vi "Induction Range Bit Pack Parse.vi"(10 "Raw Data":string, 11 "Boolean array":bool[](array[boolean])) -> (3 "String":string)   [LabVIEW 2016]
uses:
  <vilib>/Utility/error.llb/whitespace.ctl
panel:
  out "Error Out":errorcluster
  in  "Error In":errorcluster
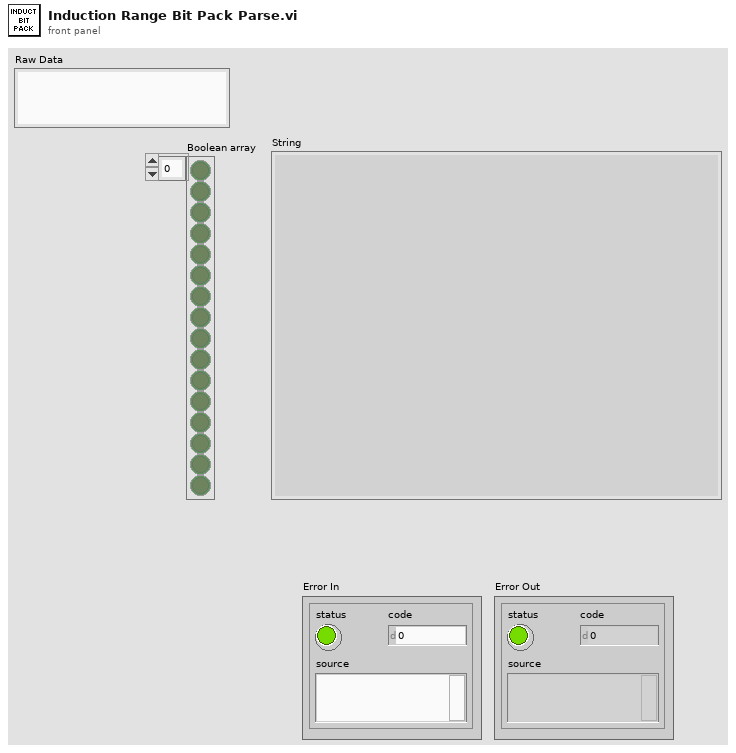
[diagram p1: front panel]
types:
  T1 = typedef "whitespace.ctl" = u16
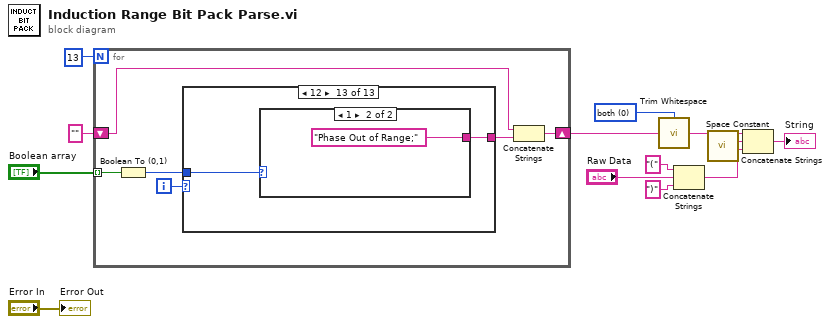
[diagram p0: block diagram]
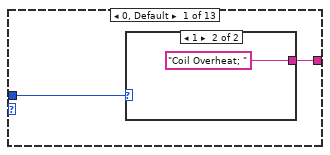
[diagram p2: hidden frame]
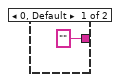
[diagram p3: hidden frame]
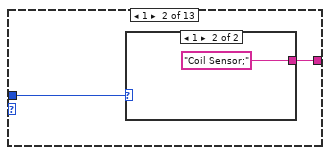
[diagram p4: hidden frame]
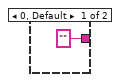
[diagram p5: hidden frame]
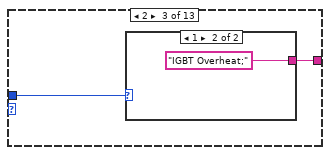
[diagram p6: hidden frame]
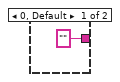
[diagram p7: hidden frame]
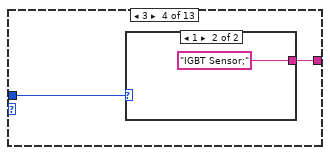
[diagram p8: hidden frame]
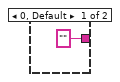
[diagram p9: hidden frame]
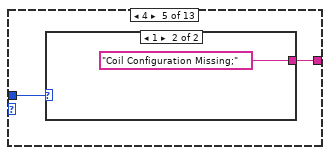
[diagram p10: hidden frame]
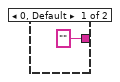
[diagram p11: hidden frame]
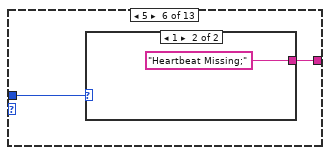
[diagram p12: hidden frame]
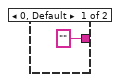
[diagram p13: hidden frame]
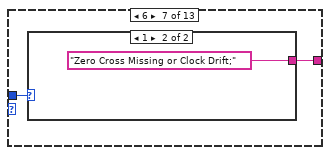
[diagram p14: hidden frame]
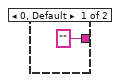
[diagram p15: hidden frame]
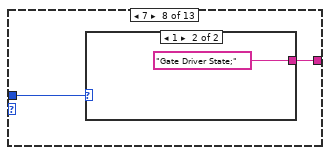
[diagram p16: hidden frame]
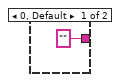
[diagram p17: hidden frame]
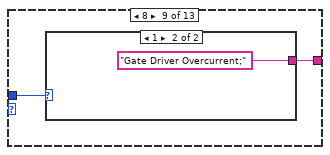
[diagram p18: hidden frame]
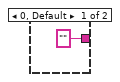
[diagram p19: hidden frame]
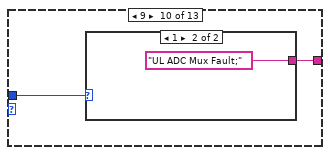
[diagram p20: hidden frame]
diagram:
  w8 = T1 0 items=["both", "start of string", "end of string"] ("location (both)")
  n1 = for {
    N: 13 -> [_]
    tunnel: "Boolean array" -> [w17] mode=indexing
    shift-right: [w18] -> w9
    shift-left: "" -> [w19]
    i -> [w16]
    n2 = Boolean To (0,1)(Boolean=w17) -> (0, 1=w15:i16)
    n3 = case shown="12" w16 {
      tunnel: w15 -> [w21 w24 w29 w32 w37 w40 w44 w48 w52 w56 w60 w64 w69]
      tunnel: [w20 w25 w28 w33 w36 w41 w45 w49 w53 w57 w61 w65 w68] -> w14
      frame 0, Default {
        n4 = case shown="1" w21 {
          tunnel: ["" "Coil Overheat; "] -> w20
          frame 0, Default {
          }
          frame 1 {
          }
        }
      }
      frame 1 {
        n5 = case shown="1" w24 {
          tunnel: ["" "Coil Sensor;"] -> w25
          frame 0, Default {
          }
          frame 1 {
          }
        }
      }
      frame 2 {
        n6 = case shown="1" w29 {
          tunnel: ["" "IGBT Overheat;"] -> w28
          frame 0, Default {
          }
          frame 1 {
          }
        }
      }
      frame 3 {
        n7 = case shown="1" w32 {
          tunnel: ["" "IGBT Sensor;"] -> w33
          frame 0, Default {
          }
          frame 1 {
          }
        }
      }
      frame 4 {
        n8 = case shown="1" w37 {
          tunnel: ["" "Coil Configuration Missing;"] -> w36
          frame 0, Default {
          }
          frame 1 {
          }
        }
      }
      frame 5 {
        n9 = case shown="1" w40 {
          tunnel: ["" "Heartbeat Missing;"] -> w41
          frame 0, Default {
          }
          frame 1 {
          }
        }
      }
      frame 6 {
        n10 = case shown="1" w44 {
          tunnel: ["" "Zero Cross Missing or Clock Drift;"] -> w45
          frame 0, Default {
          }
          frame 1 {
          }
        }
      }
      frame 7 {
        n11 = case shown="1" w48 {
          tunnel: ["" "Gate Driver State;"] -> w49
          frame 0, Default {
          }
          frame 1 {
          }
        }
      }
      frame 8 {
        n12 = case shown="1" w52 {
          tunnel: ["" "Gate Driver Overcurrent;"] -> w53
          frame 0, Default {
          }
          frame 1 {
          }
        }
      }
      frame 9 {
        n13 = case shown="1" w56 {
          tunnel: ["" "UL ADC Mux Fault;"] -> w57
          frame 0, Default {
          }
          frame 1 {
          }
        }
      }
      frame 10 {
        n14 = case shown="1" w60 {
          tunnel: ["" "Coil Current Out of Range;"] -> w61
          frame 0, Default {
          }
          frame 1 {
          }
        }
      }
      frame 11 {
        n15 = case shown="1" w64 {
          tunnel: ["" "Line Voltage Out of Range;"] -> w65
          frame 0, Default {
          }
          frame 1 {
          }
        }
      }
      frame 12 {
        n16 = case shown="1" w69 {
          tunnel: ["" "Phase Out of Range;"] -> w68
          frame 0, Default {
          }
          frame 1 {
          }
        }
      }
    }
    n17 = Concatenate Strings(w19, w14) -> (w18:string)
  }
  n18 = call <vilib>:"Trim Whitespace.vi"("string"=w9, "location (both)"=w8) -> ("trimmed string"=w4:string)
  n19 = Concatenate Strings("(" ("string"), "Raw Data", ")" ("string")) -> (w2:string)
  n20 = call <vilib>:"Space Constant.vi"() -> ("String"=w3:string)
  n21 = Concatenate Strings(w4, w3, w2) -> (→"String":string)
  "Error Out" <- "Error In"
